vi "FlipFlop.vi"() -> ()   [LabVIEW 2012]
panel:
  in  "CntEn":bool
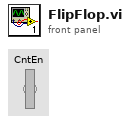
[diagram p1: front panel]
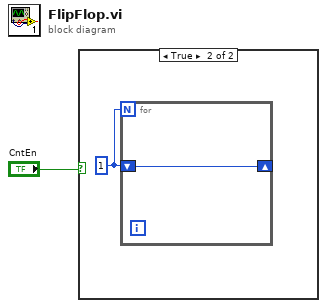
[diagram p0: block diagram]
diagram:
  n1 = case shown="True" "CntEn" {
    frame False {
    }
    frame True {
      w2 = 1
      n2 = for {
        N: w2 -> [_]
        shift-right: [w3] -> _
        shift-left: w2 -> [w3]
      }
    }
  }
